vi "quiz 3.1.vi"() -> ()   [LabVIEW 2017]
panel:
  out "unsigned byte array":u8[](array[numeric])
  out "Tab Control":T1(tab)
  in  "Ingresar":bool
  in  "usuario":string
  in  "Contraseña":string
  in  "eliminar":bool
  in  "agregar":bool
  in  "añadir":bool
  in  "contraseña":string
  in  "usuario":string
  in  "Quitar":bool
  in  "usuario a eliminar":string
  # "¿QUE DESEA REALIZAR?"
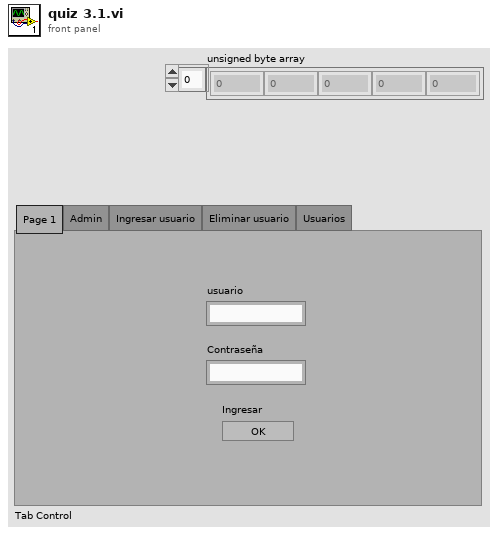
[diagram p1: front panel]
types:
  T1 = enum32{"Page 1", "Admin", "Ingresar usuario", "Eliminar usuario", "Usuarios"}
  T2 = enum16{"open", "replace", "create", "open or create", "replace or create", "replace or create with confirmation"}
  T3 = enum32{"Page 1", "Admin", "Ingresar usuario", "Eliminar usuario"}
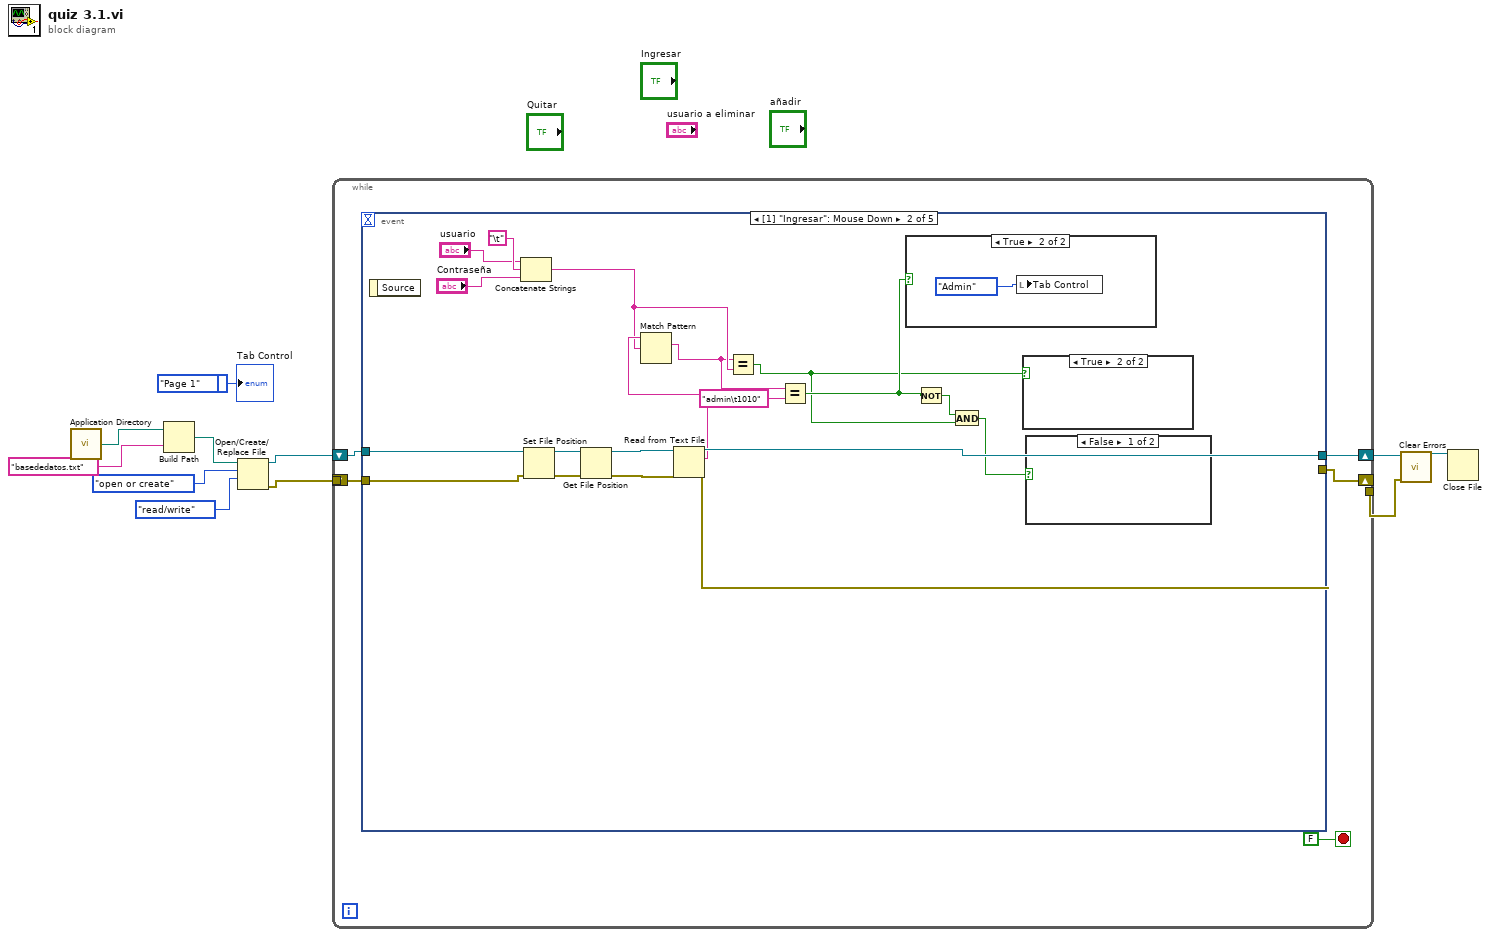
[diagram p0: block diagram]
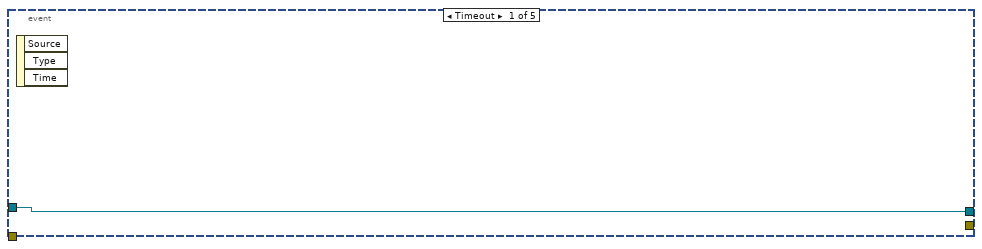
[diagram p2: hidden frame]
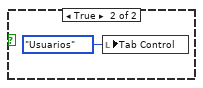
[diagram p3: hidden frame]
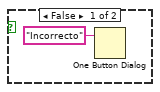
[diagram p4: hidden frame]
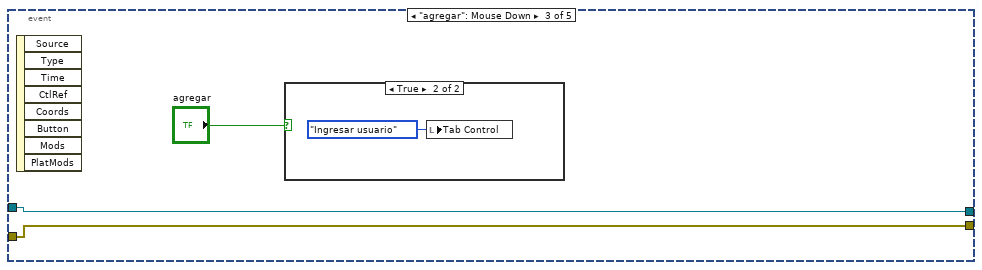
[diagram p6: hidden frame]
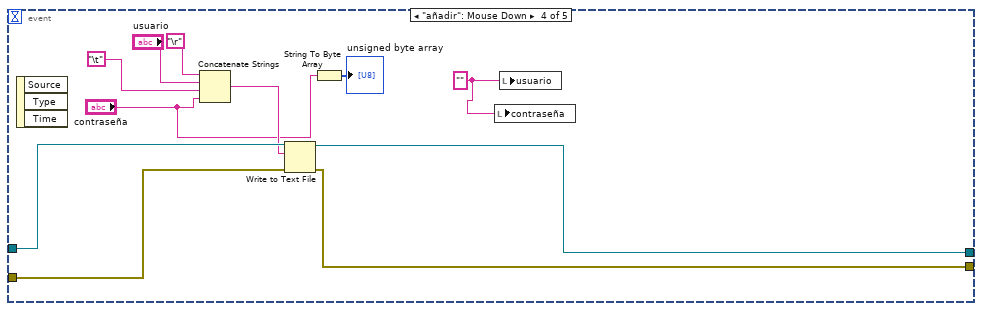
[diagram p8: hidden frame]
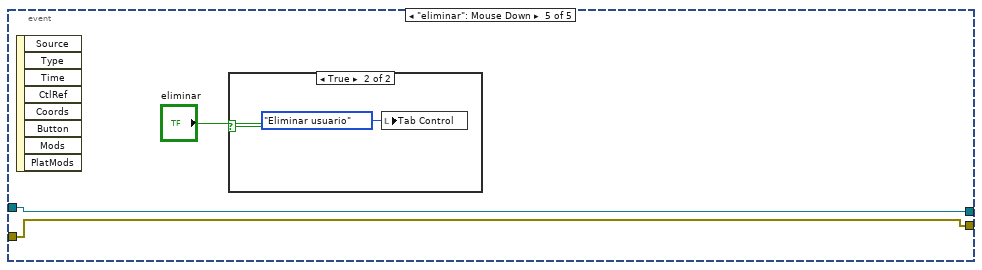
[diagram p9: hidden frame]
diagram:
  (unwired) T1."Page 1" ("Tab Control")
  n1 = call <vilib>:"Application Directory.vi"() -> ("Application Directory"=w6:path)
  n2 = Build Path(base path=w6, name or relative path="basededatos.txt") -> (appended path=w7:path)
  n3 = Open/Create/Replace File(file path (use dialog)=w7, operation (0:open)=T2."open or create", access (0:read/write)=enum16{"read/write", "read-only", "write-only"}."read/write") -> (refnum out=w3:refnum<file>, error out=w2:errorcluster)  [unwired: 3 in, 1 out]
  n4 = call <vilib>:"Clear Errors.vi"() -> ("error out"=w1:errorcluster)  [unwired: 6 in, 1 out]
  n5 = while {
    tunnel: w2 -> [w15]
    shift-right: [w14] -> w8
    shift-left: w3 -> [w12]
    shift-right: [w11] -> _
    shift-left: _ -> [_]
    tunnel: w1 -> [_]
    stop <- FALSE stop-if-true
    n6 = event shown="[1] \"Ingresar\": Mouse Down" {
      selector: _ -> [_ _ _ _ _]
      dyn-events: _ -> [_ _ _ _ _]
      timeout: _ -> [_ _ _ _ _]
      tunnel: w12 -> [w16 w31 w40 w52 w55]
      tunnel: w15 -> [_ w30 w39 w53 w54]
      tunnel: [w16 w29 w40 w51 w55] -> w14
      tunnel: [_ w25 w39 w43 w54] -> w11
      event Timeout {
        n7 = event-data() -> ()  [unwired: 1 in, 3 out]
      }
      event "Ingresar": Mouse Down {
        n8 = event-data() -> ()  [unwired: 1 in, 1 out]
        n9 = Concatenate Strings("usuario", "\t", "Contraseña") -> (w23:string)
        n10 = Set File Position(refnum=w31, error in=w30) -> (refnum out=w35:refnum<file>, error out=w33:errorcluster)  [unwired: 2 in]
        n11 = Get File Position(4:w33, 7:w35) -> (0:w32:errorcluster, 3:w34:refnum<file>)  [unwired: 1 out]
        n12 = Read from Text File(file (use dialog)=w34, error in=w32) -> (refnum out=w29:refnum<file>, text=w24:string, error out=w25:errorcluster)  [unwired: 2 in, 1 out]
        n13 = Match Pattern(string=w24, regular expression=w23) -> (match substring=w22:string)  [unwired: 1 in, 3 out]
        n14 = Equal?(x=w22, y=w23) -> (x = y?=w18:bool)
        n15 = Equal?(x=w22, y="admin\t1010") -> (x = y?=w20:bool)
        n16 = case shown="True" w20 {
          frame False {
          }
          frame True {
            n17 = local write "Tab Control"(enum32{"Page 1", "Admin", "Ingresar usuario"}."Admin" ("Tab Control")) -> ()
          }
        }
        n18 = Not(x=w20) -> (.not. x?=w19:bool)
        n19 = And(x=w19, y=w18) -> (x .and. y?=w17:bool)
        n20 = case shown="True" w18 {
          frame False {
            n21 = One Button Dialog(message="Incorrecto") -> ()  [unwired: 1 in, 1 out]
          }
          frame True {
          }
        }
        n22 = case shown="False" w17 {
          frame False {
          }
          frame True {
            n23 = local write "Tab Control"(T1."Usuarios" ("Tab Control")) -> ()
          }
        }
      }
      event "agregar": Mouse Down {
        n24 = event-data() -> ()  [unwired: 1 in, 8 out]
        n25 = case shown="True" "agregar" {
          frame False {
          }
          frame True {
            n26 = local write "Tab Control"(enum32{"Page 1", "Admin", "Ingresar usuario"}."Ingresar usuario" ("Tab Control")) -> ()
          }
        }
      }
      event "añadir": Mouse Down {
        w46 = "" ("usuario")
        n27 = event-data() -> ()  [unwired: 1 in, 3 out]
        n28 = Concatenate Strings("\r", "usuario", "\t", "contraseña") -> (w49:string)
        n29 = Write to Text File(file (use dialog)=w52, text=w49, error in=w53) -> (refnum out=w51:refnum<file>, error out=w43:errorcluster)  [unwired: 1 in, 1 out]
        n30 = String To Byte Array(string="contraseña") -> (unsigned byte array=→"unsigned byte array":u8[])
        n31 = local write "contraseña"(w46) -> ()
        n32 = local write "usuario"(w46) -> ()
      }
      event "eliminar": Mouse Down {
        n33 = event-data() -> ()  [unwired: 1 in, 8 out]
        n34 = case shown="True" "eliminar" {
          frame False {
          }
          frame True {
            n35 = local write "Tab Control"(T3."Eliminar usuario" ("Tab Control")) -> ()
          }
        }
      }
    }
  }
  n36 = Close File(refnum=w8) -> ()  [unwired: 1 in, 2 out]
  "Tab Control" <- enum32{"Page 1", "Admin", "Ingresar usuario"}."Page 1" ("Tab Control")
